vi "Resample Array of Pairs (single shot).vi"(0 "XY-data in":cluster{"x":dbl, "y":dbl}[](array[cluster]) {"y" format="%.2p"; "x" format="%.2p"}, 5 "dt":dbl=1.0 format="%.2p", 7 "t0":dbl=-inf format="%.2p", 9 "interpolation mode":u16(ring)=1 items=["coerce", "linear", "spline", "FIR filter"], 11 "error in (no error)":errorcluster) -> (4 "resampled waveform out":waveform(dbl), 6 "XY-data out":cluster{"x":dbl, "y":dbl}[](array[cluster]) {"y" format="%.2p"; "x" format="%.2p"}, 10 "used t0":dbl format="%.2p", 14 "t0 adjusted warning":bool, 15 "error out":errorcluster)   [LabVIEW 2020, in "NI_MAPro.lvlib"]
doc: "Resamples input waveforms or data according to the user-defined <B>t0</B> and <B>dt</B> values.\n\nWire data to the waveform or data input to determine the polymorphic instance to use or manually select the instance."
uses:
  NI_MAPro.lvlib
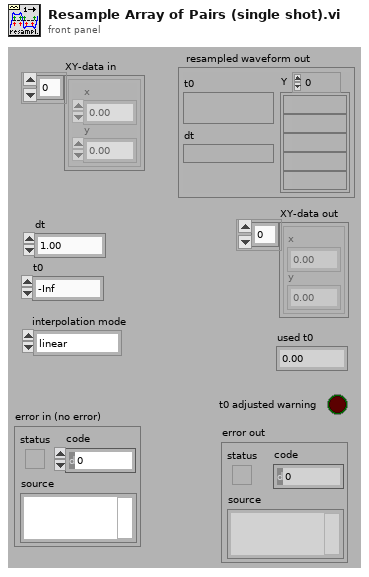
[diagram p1: front panel]
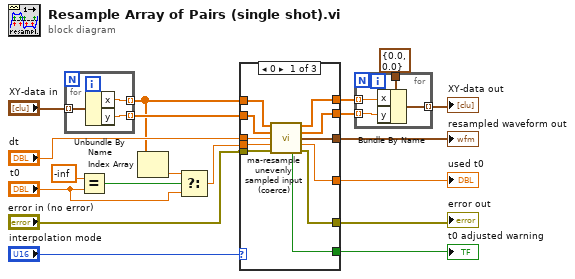
[diagram p0: block diagram]
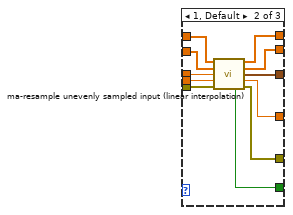
[diagram p2: hidden frame]
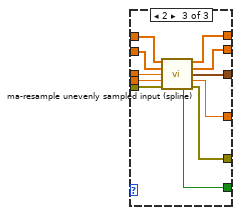
[diagram p3: hidden frame]
diagram:
  n1 = for {
    tunnel: "XY-data in" -> [w22] mode=indexing
    tunnel: [w21] -> w6 mode=indexing
    tunnel: [w20] -> w9 mode=indexing
    n2 = Unbundle By Name(w22) -> ("x"=w21:dbl, "y"=w20:dbl)
  }
  n3 = Equal?(x=-inf, y="t0") -> (x = y?=w17:bool)
  n4 = Index Array(array=w6) -> (element=w7:dbl)  [unwired: 1 in]
  n5 = Select(t=w7, s=w17, f="t0") -> (s? t:f=w15:dbl)
  n6 = case shown="0" "interpolation mode" {
    tunnel: "error in (no error)" -> [w33 w44 w55]
    tunnel: "dt" -> [w32 w43 w54]
    tunnel: w15 -> [w31 w42 w53]
    tunnel: [w30 w41 w52] -> w14
    tunnel: [w29 w40 w51] -> w13
    tunnel: [w28 w39 w50] -> w12
    tunnel: [w27 w38 w49] -> w11
    tunnel: w6 -> [w24 w37 w46]
    tunnel: w9 -> [w23 w36 w45]
    tunnel: [w26 w35 w48] -> w3
    tunnel: [w25 w34 w47] -> w4
    frame 0 {
      n7 = call "ma-resample unevenly sampled input (coerce).vi"("X-array in"=w24, "Y-array in"=w23, "dt"=w32, "t0"=w31, "error in"=w33) -> ("X-array out"=w25:dbl[], "Y-array out"=w26:dbl[], "evenly sampled waveform out"=w27:waveform(dbl), "used t0"=w28:dbl, "t0 adjusted warning"=w30:bool, "error out"=w29:errorcluster)  [unwired: 5 in]
    }
    frame 1, Default {
      n8 = call "ma-resample unevenly sampled input (linear interpolation).vi"("X-array in"=w37, "Y-array in"=w36, "dt"=w43, "t0"=w42, "error in"=w44) -> ("X-array out"=w34:dbl[], "Y-array out"=w35:dbl[], "evenly sampled waveform out"=w38:waveform(dbl), "used t0"=w39:dbl, "t0 adjusted warning"=w41:bool, "error out"=w40:errorcluster)  [unwired: 5 in]
    }
    frame 2 {
      n9 = call "ma-resample unevenly sampled input (spline).vi"("X-array in"=w46, "Y-array in"=w45, "dt"=w54, "t0"=w53, "error in"=w55) -> ("X-array out"=w47:dbl[], "Y-array out"=w48:dbl[], "evenly sampled waveform out"=w49:waveform(dbl), "used t0"=w50:dbl, "t0 adjusted warning"=w52:bool, "error out"=w51:errorcluster)  [unwired: 5 in]
    }
  }
  "error out" <- w13
  "t0 adjusted warning" <- w14
  "used t0" <- w12
  "resampled waveform out" <- w11
  n10 = for {
    tunnel: cluster{"x":dbl, "y":dbl} {"x"=0.0, "y"=0.0} -> [w59]
    tunnel: w4 -> [w58] mode=indexing
    tunnel: w3 -> [w57] mode=indexing
    tunnel: [w56] -> w2 mode=indexing
    n11 = Bundle By Name(cluster=w59, "x"=w58, "y"=w57) -> (w56:cluster{"x":dbl, "y":dbl})
  }
  "XY-data out" <- w2
